vi "打开连接.vi"(11 "IP Address":string="10.0.0.5") -> (0 "error out":errorcluster, 3 "TCP Connection Ref":refnum<k5>)   [LabVIEW 2017]
uses:
  S7 TCP API Library/S7 TCP.lvlib
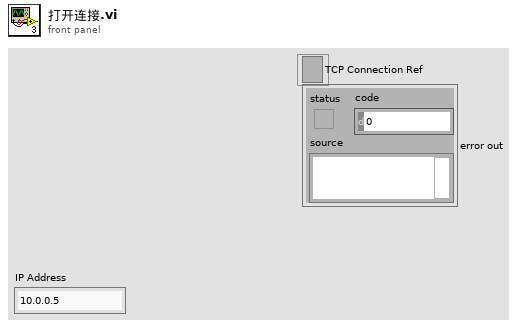
[diagram p1: front panel]
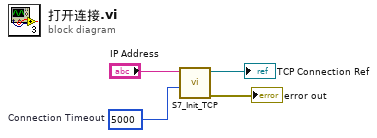
[diagram p0: block diagram]
diagram:
  w4 = u32 5000  # Connection Timeout
  n1 = call "S7_Init_TCP.vi"("Connection Timeout"=w4, "IP Address"="IP Address") -> ("error out"=→"error out":errorcluster, "TCP Connection Ref"=→"TCP Connection Ref":refnum<k5>)  [unwired: 3 in, 5 out]
